vi "input.vi"(8 "error in":errorcluster, 10 "data table in":T5, 11 "SystemLin Tag Module runtime in":refnum<class "SystemLink File runtime.lvclass">) -> (0 "error out":errorcluster, 2 "data table out":T5, 3 "SystemLin Tag Module runtime out":refnum<class "SystemLink File runtime.lvclass">)   [LabVIEW 2015]
doc: "Provides an interface for reading data from a module at runtime. While this interface performs no operations, a child should provide an override which may read from any open sessions, references, or interfaces."
uses:
  <vilib>/NI/Tag Bus/table/data table.lvlib
  <vilib>/NI/Tag Bus/table/data polymorphs/write one/write Double.vi
  <vilib>/NI/Tag Bus/table/data polymorphs/write one/write Single.vi
  <vilib>/NI/Tag Bus/table/data polymorphs/write one/write I32.vi
  <vilib>/NI/Tag Bus/table/data polymorphs/write one/write I16.vi
  <vilib>/NI/Tag Bus/table/data polymorphs/write one/write I8.vi
  <vilib>/NI/Tag Bus/table/data polymorphs/write one/write Boolean.vi
  <vilib>/Skyline/Tag/Wrapper/Wrapper_class/NI Skyline Tag.lvclass
  <vilib>/Skyline/Tag/Wrapper/Wrapper_class/Read Tag (I32).vi
  <vilib>/Skyline/Tag/Wrapper/Wrapper_class/Read Tag (DBL).vi
  <vilib>/Skyline/Tag/Wrapper/Wrapper_class/Read Tag (String).vi
  <vilib>/NI/Tag Bus/table/data polymorphs/write one/write String.vi
  <vilib>/NI/Tag Bus/table/data polymorphs/write one/write U64.vi
  <vilib>/Skyline/Tag/Wrapper/Wrapper_class/Read Tag (Boolean).vi
  <vilib>/Skyline/Tag/Wrapper/Wrapper_class/Read Tag (U64).vi
  <vilib>/NI/Tag Bus/table/data polymorphs/write one/write U32.vi
  <vilib>/NI/Tag Bus/table/data polymorphs/write one/write U16.vi
  <vilib>/NI/Tag Bus/table/data polymorphs/write one/write U8.vi
  <vilib>/Skyline/Tag/Wrapper/Wrapper_class/Read Tag (Timestamp).vi
  SystemLink File runtime.lvclass
  <vilib>/NI/Tag Bus/table/data table.ctl
  <vilib>/Skyline/Tag/Shared/typedefs/DataType.ctl
  <vilib>/Skyline/Tag/Shared/NI Skyline Tag.lvlib
  <vilib>/Skyline/Tag/Shared/typedefs/Tag Value Cluster.ctl
  configuration/SysLink Mapping.ctl
  configuration/SystemLink File configuration.lvclass
  configuration/Data Tag Type.ctl
panel:
  out "Inputs Array":refnum<class "NI Skyline Tag.lvclass">[](array[class])
  out "Input Map":T1[](array[typedef])
  out "tag clusters":T3[](array[typedef])
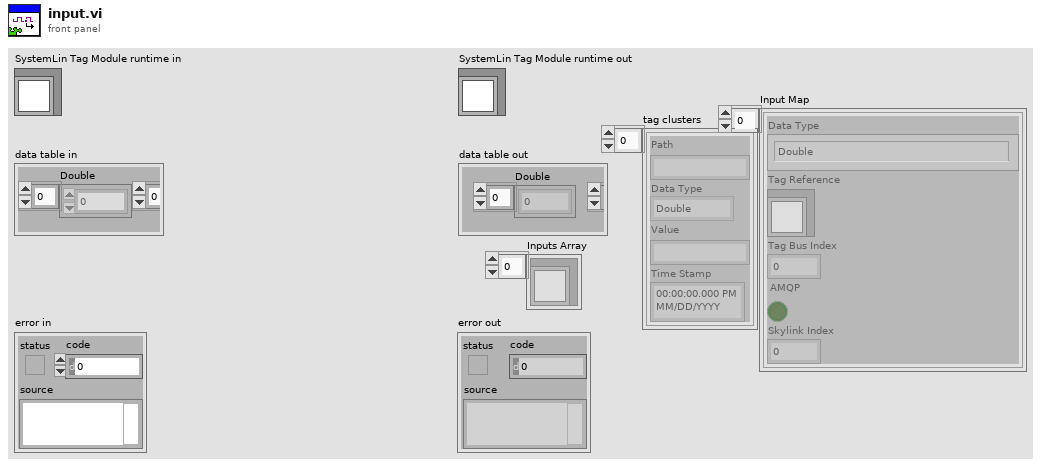
[diagram p1: front panel]
types:
  T1 = typedef "SystemLink File configuration.lvclass/SysLink Mapping.ctl" = cluster{"Data Type":T2, "Tag Reference":refnum<class "NI Skyline Tag.lvclass">, "Tag Bus Index":i32, "AMQP":bool, "Skylink Index":i32}
  T2 = typedef "SystemLink File configuration.lvclass/Data Tag Type.ctl" = enum16{"Double", "Single", "I32", "I16", "I8", "U64", "U32", "U16", "U8", "Boolean", "String", "Timestamp"}
  T3 = typedef "NI Skyline Tag.lvlib/Tag Value Cluster.ctl" = cluster{"Path":string, "Data Type":T4, "Value":string, "Time Stamp":timestamp}
  T4 = typedef "NI Skyline Tag.lvlib/DataType.ctl" = enum32{"Double", "I32", "String", "Boolean", "U64", "Timestamp"}
  T5 = typedef "tag bus.lvlib/data table.lvlib/data table.ctl" = cluster{"Double":dbl[], "Single":sgl[], "I64":i64[], "I32":i32[], "I16":i16[], "I8":i8[], "U64":u64[], "U32":u32[], "U16":u16[], "U8":u8[], "Boolean":bool[], "String":string[], "Array of Double":cluster{"DBL Array":dbl[]}[], "Array of Single":cluster{"SGL Array":sgl[]}[], "Array of I64":cluster{"I64 Array":i64[]}[], "Array of I32":cluster{"I32 Array":i32[]}[], "Array of I16":cluster{"I16 Array":i16[]}[], "Array of I8":cluster{"I8 Array":i8[]}[], "Array of U64":cluster{"U64 Array":u64[]}[], "Array of U32":cluster{"U32 Array":u32[]}[], "Array of U16":cluster{"U16 Array":u16[]}[], "Array of U8":cluster{"U8 Array":u8[]}[], "Array of Boolean":cluster{"Boolean Array":bool[]}[], "Array of String":cluster{"String Array":string[]}[]}
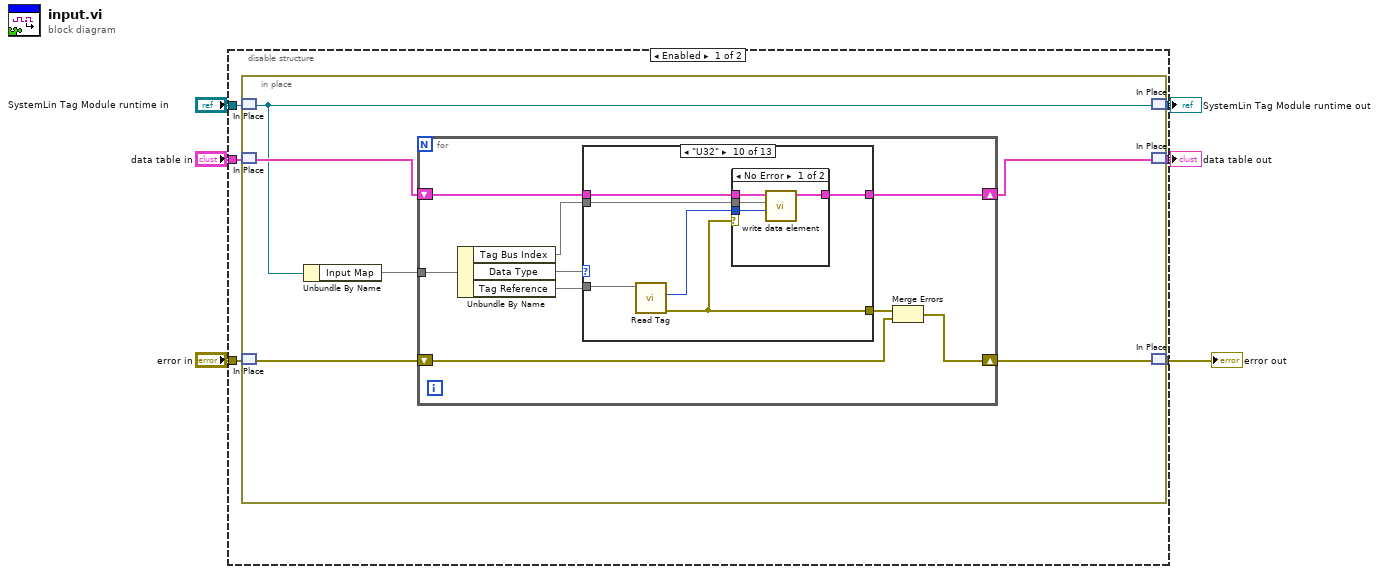
[diagram p0: block diagram]
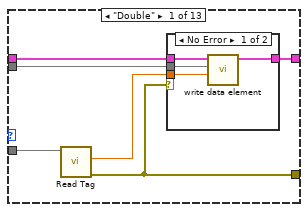
[diagram p2: hidden frame]
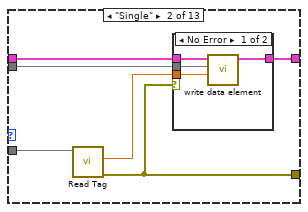
[diagram p4: hidden frame]
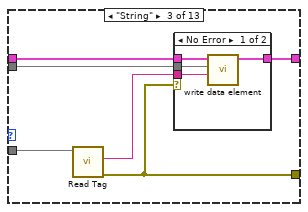
[diagram p6: hidden frame]
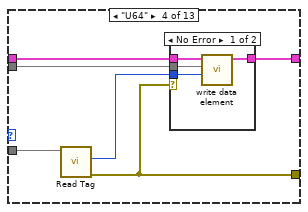
[diagram p8: hidden frame]
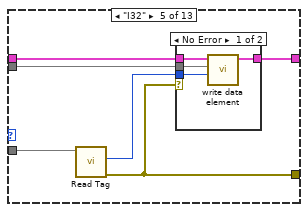
[diagram p10: hidden frame]
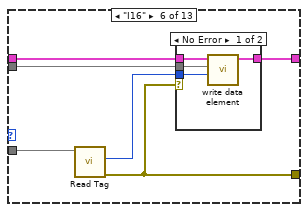
[diagram p12: hidden frame]
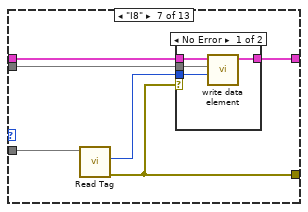
[diagram p14: hidden frame]
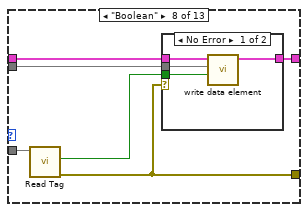
[diagram p16: hidden frame]
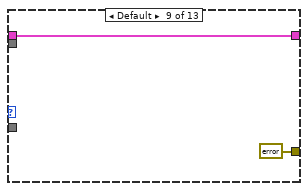
[diagram p18: hidden frame]
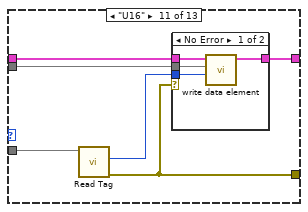
[diagram p20: hidden frame]
diagram:
  n1 = disable-structure shown="Enabled" {
    disable-tunnel: "SystemLin Tag Module runtime in" -> [w12 w168]
    disable-tunnel: [w11 w167] -> w5
    disable-tunnel: "data table in" -> [w10 w166]
    disable-tunnel: [w9 w165] -> w3
    disable-tunnel: [w8 w164] -> w2
    disable-tunnel: "error in" -> [w7 w163]
    frame Enabled {
      n2 = in-place {
        n3 = in-place-match #1(w12) -> (w14:refnum<class "SystemLink File runtime.lvclass">)
        n4 = in-place-match #2(w10) -> (w18:T5)
        n5 = in-place-match #3(w7) -> (w16:errorcluster)
        n6 = Unbundle By Name(w14) -> ("Input Map"=w13)
        n7 = for {
          shift-right: [w24] -> w17
          shift-left: w18 -> [w25]
          shift-right: [w21] -> w15
          shift-left: w16 -> [w20]
          tunnel: w13 -> [w27]
          n8 = Unbundle By Name(w27) -> ("Tag Bus Index"=w23, "Data Type"=w26, "Tag Reference"=w19)
          n9 = case shown="\"U32\"" w26 {
            tunnel: w25 -> [w33 w44 w55 w64 w77 w88 w99 w110 w117 w122 w133 w144 w156]
            tunnel: [w32 w43 w54 w65 w76 w87 w98 w109 w117 w123 w134 w145 w157] -> w24
            tunnel: w23 -> [w31 w42 w53 w63 w75 w86 w97 w108 _ w119 w132 w143 w155]
            tunnel: w19 -> [w30 w41 w52 w66 w74 w85 w96 w107 _ w120 w131 w142 w154]
            tunnel: [w28 w39 w50 w61 w72 w83 w94 w106 errorcluster {"status"=FALSE, "code"=0, "source"=""} ("error IO") w121 w129 w141 w151] -> w22
            frame "Double" {
              n10 = call-poly <vilib>:"Read Tag.vi"("tag in"=w30) -> ("error out"=w28:errorcluster, "value"=w29:dbl)  [unwired: 6 in, 3 out]
              n11 = case shown="No Error" w28 {
                tunnel: w33 -> [w37 w38]
                tunnel: [w36 w38] -> w32
                tunnel: w31 -> [w35 _]
                tunnel: w29 -> [w34 _]
                frame No Error {
                  n12 = call-poly <vilib>:"write data element.vi"("value"=w34, "index"=w35, "data table in"=w37) -> ("data table out"=w36:T5)  [unwired: 8 in]
                }
                frame Error {
                }
              }
            }
            frame "Single" {
              n13 = call-poly <vilib>:"Read Tag.vi"("tag in"=w41) -> ("error out"=w39:errorcluster, "value"=w40:dbl)  [unwired: 6 in, 3 out]
              n14 = case shown="No Error" w39 {
                tunnel: w44 -> [w48 w49]
                tunnel: [w47 w49] -> w43
                tunnel: w42 -> [w46 _]
                tunnel: w40 -> [w45 _]
                frame No Error {
                  n15 = call-poly <vilib>:"write data element.vi"("value"=w45, "index"=w46, "data table in"=w48) -> ("data table out"=w47:T5)  [unwired: 8 in]
                }
                frame Error {
                }
              }
            }
            frame "String" {
              n16 = call-poly <vilib>:"Read Tag.vi"("tag in"=w52) -> ("error out"=w50:errorcluster, "value"=w51:string)  [unwired: 6 in, 3 out]
              n17 = case shown="No Error" w50 {
                tunnel: w55 -> [w59 w60]
                tunnel: [w58 w60] -> w54
                tunnel: w53 -> [w57 _]
                tunnel: w51 -> [w56 _]
                frame No Error {
                  n18 = call-poly <vilib>:"write data element.vi"("value"=w56, "index"=w57, "data table in"=w59) -> ("data table out"=w58:T5)  [unwired: 8 in]
                }
                frame Error {
                }
              }
            }
            frame "U64" {
              n19 = call-poly <vilib>:"Read Tag.vi"("tag in"=w66) -> ("error out"=w61:errorcluster, "value"=w62:u64)  [unwired: 6 in, 3 out]
              n20 = case shown="No Error" w61 {
                tunnel: w64 -> [w70 w71]
                tunnel: [w69 w71] -> w65
                tunnel: w63 -> [w68 _]
                tunnel: w62 -> [w67 _]
                frame No Error {
                  n21 = call-poly <vilib>:"write data element.vi"("value"=w67, "index"=w68, "data table in"=w70) -> ("data table out"=w69:T5)  [unwired: 8 in]
                }
                frame Error {
                }
              }
            }
            frame "I32" {
              n22 = call-poly <vilib>:"Read Tag.vi"("tag in"=w74) -> ("error out"=w72:errorcluster, "value"=w73:i32)  [unwired: 6 in, 3 out]
              n23 = case shown="No Error" w72 {
                tunnel: w77 -> [w81 w82]
                tunnel: [w80 w82] -> w76
                tunnel: w75 -> [w79 _]
                tunnel: w73 -> [w78 _]
                frame No Error {
                  n24 = call-poly <vilib>:"write data element.vi"("value"=w78, "index"=w79, "data table in"=w81) -> ("data table out"=w80:T5)  [unwired: 8 in]
                }
                frame Error {
                }
              }
            }
            frame "I16" {
              n25 = call-poly <vilib>:"Read Tag.vi"("tag in"=w85) -> ("error out"=w83:errorcluster, "value"=w84:i32)  [unwired: 6 in, 3 out]
              n26 = case shown="No Error" w83 {
                tunnel: w88 -> [w92 w93]
                tunnel: [w91 w93] -> w87
                tunnel: w86 -> [w90 _]
                tunnel: w84 -> [w89 _]
                frame No Error {
                  n27 = call-poly <vilib>:"write data element.vi"("value"=w89, "index"=w90, "data table in"=w92) -> ("data table out"=w91:T5)  [unwired: 8 in]
                }
                frame Error {
                }
              }
            }
            frame "I8" {
              n28 = call-poly <vilib>:"Read Tag.vi"("tag in"=w96) -> ("error out"=w94:errorcluster, "value"=w95:i32)  [unwired: 6 in, 3 out]
              n29 = case shown="No Error" w94 {
                tunnel: w99 -> [w103 w104]
                tunnel: [w102 w104] -> w98
                tunnel: w97 -> [w101 _]
                tunnel: w95 -> [w100 _]
                frame No Error {
                  n30 = call-poly <vilib>:"write data element.vi"("value"=w100, "index"=w101, "data table in"=w103) -> ("data table out"=w102:T5)  [unwired: 8 in]
                }
                frame Error {
                }
              }
            }
            frame "Boolean" {
              n31 = call-poly <vilib>:"Read Tag.vi"("tag in"=w107) -> ("error out"=w106:errorcluster, "value"=w105:bool)  [unwired: 6 in, 3 out]
              n32 = case shown="No Error" w106 {
                tunnel: w110 -> [w114 w115]
                tunnel: [w113 w115] -> w109
                tunnel: w108 -> [w112 _]
                tunnel: w105 -> [w111 _]
                frame No Error {
                  n33 = call-poly <vilib>:"write data element.vi"("value"=w111, "index"=w112, "data table in"=w114) -> ("data table out"=w113:T5)  [unwired: 8 in]
                }
                frame Error {
                }
              }
            }
            frame Default {
            }
            frame "U32" {
              n34 = call-poly <vilib>:"Read Tag.vi"("tag in"=w120) -> ("error out"=w121:errorcluster, "value"=w118:u64)  [unwired: 6 in, 3 out]
              n35 = case shown="No Error" w121 {
                tunnel: w122 -> [w127 w128]
                tunnel: [w126 w128] -> w123
                tunnel: w119 -> [w125 _]
                tunnel: w118 -> [w124 _]
                frame No Error {
                  n36 = call-poly <vilib>:"write data element.vi"("value"=w124, "index"=w125, "data table in"=w127) -> ("data table out"=w126:T5)  [unwired: 8 in]
                }
                frame Error {
                }
              }
            }
            frame "U16" {
              n37 = call-poly <vilib>:"Read Tag.vi"("tag in"=w131) -> ("error out"=w129:errorcluster, "value"=w130:u64)  [unwired: 6 in, 3 out]
              n38 = case shown="No Error" w129 {
                tunnel: w133 -> [w138 w139]
                tunnel: [w137 w139] -> w134
                tunnel: w132 -> [w136 _]
                tunnel: w130 -> [w135 _]
                frame No Error {
                  n39 = call-poly <vilib>:"write data element.vi"("value"=w135, "index"=w136, "data table in"=w138) -> ("data table out"=w137:T5)  [unwired: 8 in]
                }
                frame Error {
                }
              }
            }
            frame "U8" {
              n40 = call-poly <vilib>:"Read Tag.vi"("tag in"=w142) -> ("error out"=w141:errorcluster, "value"=w140:u64)  [unwired: 6 in, 3 out]
              n41 = case shown="No Error" w141 {
                tunnel: w144 -> [w149 w150]
                tunnel: [w148 w150] -> w145
                tunnel: w143 -> [w147 _]
                tunnel: w140 -> [w146 _]
                frame No Error {
                  n42 = call-poly <vilib>:"write data element.vi"("value"=w146, "index"=w147, "data table in"=w149) -> ("data table out"=w148:T5)  [unwired: 8 in]
                }
                frame Error {
                }
              }
            }
            frame "Timestamp" {
              n43 = call-poly <vilib>:"Read Tag.vi"("tag in"=w154) -> ("error out"=w151:errorcluster, "value"=w153:timestamp)  [unwired: 6 in, 3 out]
              n44 = To Double Precision Float(number=w153) -> (double precision float=w152:dbl)
              n45 = case shown="No Error" w151 {
                tunnel: w156 -> [w161 w162]
                tunnel: [w160 w162] -> w157
                tunnel: w155 -> [w159 _]
                tunnel: w152 -> [w158 _]
                frame No Error {
                  n46 = call-poly <vilib>:"write data element.vi"("value"=w158, "index"=w159, "data table in"=w161) -> ("data table out"=w160:T5)  [unwired: 8 in]
                }
                frame Error {
                }
              }
            }
          }
          n47 = Merge Errors(w22, w20) -> (w21:errorcluster)
        }
        n48 = in-place-match #1(w14) -> (w11:refnum<class "SystemLink File runtime.lvclass">)
        n49 = in-place-match #2(w17) -> (w9:T5)
        n50 = in-place-match #3(w15) -> (w8:errorcluster)
      }
    }
    frame Disabled {
      n51 = in-place {
        n52 = in-place-match #4(w168) -> (w174:refnum<class "SystemLink File runtime.lvclass">)
        n53 = in-place-match #5(w166) -> (w177:T5)
        n54 = in-place-match #6(w163) -> (w172:errorcluster)
        n55 = Unbundle By Name(w174) -> ("Input Map"=w173, "Inputs Array"=w170)
        "Input Map" <- w173
        "Inputs Array" <- w170
        n56 = call <vilib>:"Multi Read 2.vi"("error in (no error)"=w172, "tags in"=w170) -> ("error out"=w171:errorcluster, "tag clusters"=w169:T3[])  [unwired: 7 in, 1 out]
        "tag clusters" <- w169
        n57 = for {
          shift-right: [w184] -> w176
          shift-left: w177 -> [w185]
          shift-right: [w182] -> w175
          shift-left: w171 -> [w178]
          tunnel: w173 -> [w187]
          tunnel: w169 -> [w180] mode=indexing
          n58 = Unbundle By Name(w187) -> ("Tag Bus Index"=w183, "Data Type"=w186, "Tag Reference"=w181)
          n59 = Unbundle By Name(w180) -> ("Value"=w179:string)
          n60 = case shown="\"Double\"" w186 {
            tunnel: w185 -> [w194 w206 w216 w229 w242 w255 w268 w280 w287]
            tunnel: [w193 w205 w215 w228 w241 w254 w267 w279 w287] -> w184
            tunnel: w183 -> [w192 w204 w214 w227 w240 w253 w266 w278 _]
            tunnel: w181 -> [_ _ _ _ _ _ _ _ _]
            tunnel: [w188 w200 w212 w223 w237 w248 w263 w274 errorcluster {"status"=FALSE, "code"=0, "source"=""} ("error IO")] -> w182
            tunnel: w179 -> [w191 w203 w213 w225 w239 w252 w265 w277 _]
            tunnel: w178 -> [w190 w202 w212 w224 w238 w251 w264 w274 _]
            frame "Double" {
              n61 = Scan From String(input string=w191, error in=w190) -> (error out=w188:errorcluster, output 1=w189:dbl)  [unwired: 3 in, 2 out]
              n62 = case shown="No Error" w188 {
                tunnel: w194 -> [w198 w199]
                tunnel: [w197 w199] -> w193
                tunnel: w192 -> [w196 _]
                tunnel: w189 -> [w195 _]
                frame No Error {
                  n63 = call-poly <vilib>:"write data element.vi"("value"=w195, "index"=w196, "data table in"=w198) -> ("data table out"=w197:T5)  [unwired: 8 in]
                }
                frame Error {
                }
              }
            }
            frame "Single" {
              n64 = Scan From String(input string=w203, error in=w202) -> (error out=w200:errorcluster, output 1=w201:dbl)  [unwired: 3 in, 2 out]
              n65 = case shown="No Error" w200 {
                tunnel: w206 -> [w210 w211]
                tunnel: [w209 w211] -> w205
                tunnel: w204 -> [w208 _]
                tunnel: w201 -> [w207 _]
                frame No Error {
                  n66 = call-poly <vilib>:"write data element.vi"("value"=w207, "index"=w208, "data table in"=w210) -> ("data table out"=w209:T5)  [unwired: 8 in]
                }
                frame Error {
                }
              }
            }
            frame "String" {
              n67 = case shown="No Error" w212 {
                tunnel: w216 -> [w220 w221]
                tunnel: [w219 w221] -> w215
                tunnel: w214 -> [w218 _]
                tunnel: w213 -> [w217 _]
                frame No Error {
                  n68 = call-poly <vilib>:"write data element.vi"("value"=w217, "index"=w218, "data table in"=w220) -> ("data table out"=w219:T5)  [unwired: 8 in]
                }
                frame Error {
                }
              }
            }
            frame "I32" {
              n69 = Scan From String(input string=w225, error in=w224, default 1=0 ("value")) -> (error out=w223:errorcluster, output 1=w222:i32)  [unwired: 2 in, 2 out]
              n70 = case shown="No Error" w223 {
                tunnel: w229 -> [w233 w234]
                tunnel: [w232 w234] -> w228
                tunnel: w227 -> [w231 _]
                tunnel: w222 -> [w230 _]
                frame No Error {
                  n71 = call-poly <vilib>:"write data element.vi"("value"=w230, "index"=w231, "data table in"=w233) -> ("data table out"=w232:T5)  [unwired: 8 in]
                }
                frame Error {
                }
              }
            }
            frame "U64" {
              n72 = Scan From String(input string=w239, error in=w238, default 1=u64 0 ("value")) -> (error out=w237:errorcluster, output 1=w236:u64)  [unwired: 2 in, 2 out]
              n73 = case shown="No Error" w237 {
                tunnel: w242 -> [w246 w247]
                tunnel: [w245 w247] -> w241
                tunnel: w240 -> [w244 _]
                tunnel: w236 -> [w243 _]
                frame No Error {
                  n74 = call-poly <vilib>:"write data element.vi"("value"=w243, "index"=w244, "data table in"=w246) -> ("data table out"=w245:T5)  [unwired: 8 in]
                }
                frame Error {
                }
              }
            }
            frame "I16" {
              n75 = Scan From String(input string=w252, error in=w251, default 1=i16 0 ("value")) -> (error out=w248:errorcluster, output 1=w250:i16)  [unwired: 2 in, 2 out]
              n76 = case shown="No Error" w248 {
                tunnel: w255 -> [w259 w260]
                tunnel: [w258 w260] -> w254
                tunnel: w253 -> [w257 _]
                tunnel: w250 -> [w256 _]
                frame No Error {
                  n77 = call-poly <vilib>:"write data element.vi"("value"=w256, "index"=w257, "data table in"=w259) -> ("data table out"=w258:T5)  [unwired: 8 in]
                }
                frame Error {
                }
              }
            }
            frame "I8" {
              n78 = Scan From String(input string=w265, error in=w264, default 1=i8 0 ("value")) -> (error out=w263:errorcluster, output 1=w262:i8)  [unwired: 2 in, 2 out]
              n79 = case shown="No Error" w263 {
                tunnel: w268 -> [w272 w273]
                tunnel: [w271 w273] -> w267
                tunnel: w266 -> [w270 _]
                tunnel: w262 -> [w269 _]
                frame No Error {
                  n80 = call-poly <vilib>:"write data element.vi"("value"=w269, "index"=w270, "data table in"=w272) -> ("data table out"=w271:T5)  [unwired: 8 in]
                }
                frame Error {
                }
              }
            }
            frame "Boolean" {
              n81 = Equal?(x="True", y=w277) -> (x = y?=w275:bool)
              n82 = case shown="No Error" w274 {
                tunnel: w280 -> [w284 w285]
                tunnel: [w283 w285] -> w279
                tunnel: w278 -> [w282 _]
                tunnel: w275 -> [w281 _]
                frame No Error {
                  n83 = call-poly <vilib>:"write data element.vi"("value"=w281, "index"=w282, "data table in"=w284) -> ("data table out"=w283:T5)  [unwired: 8 in]
                }
                frame Error {
                }
              }
            }
            frame Default {
            }
          }
        }
        n84 = in-place-match #4(w174) -> (w167:refnum<class "SystemLink File runtime.lvclass">)
        n85 = in-place-match #5(w176) -> (w165:T5)
        n86 = in-place-match #6(w175) -> (w164:errorcluster)
      }
    }
  }
  "error out" <- w2
  "SystemLin Tag Module runtime out" <- w5
  "data table out" <- w3
